vi "Write loopTimer.vi"(8 "error in (no error)":errorcluster, 10 "ILoopTimer.lvclass":refnum<class "ILoopTimer.lvclass">, 11 "WindowsTarget in":refnum<class "WindowsTarget.lvclass">) -> (0 "error out":errorcluster, 3 "WindowsTarget out":refnum<class "WindowsTarget.lvclass">)   [LabVIEW 2015, in "WindowsTarget.lvclass"]
uses:
  WindowsTarget.lvclass
  ComponentTemplateCore/ComponentModel/ComponentModelRT/LoopTimer/ILoopTimer/ILoopTimer.lvclass
  WindowsTarget.lvclass/WindowsTarget.ctl
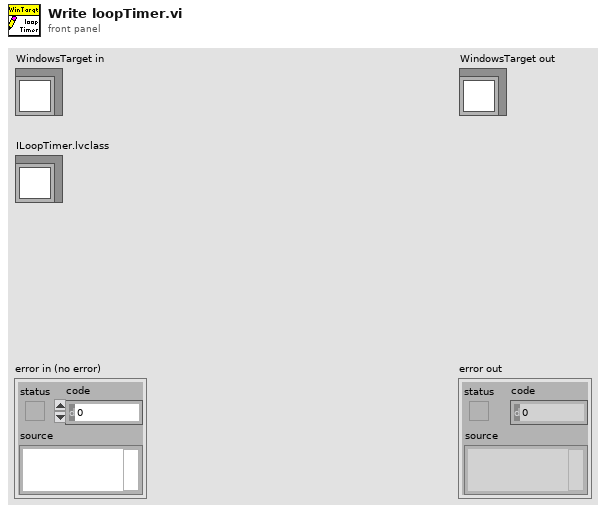
[diagram p1: front panel]
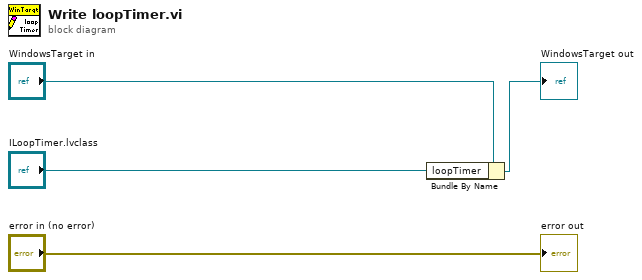
[diagram p0: block diagram]
diagram:
  n1 = Bundle By Name(cluster="WindowsTarget in", "loopTimer"="ILoopTimer.lvclass") -> (→"WindowsTarget out":refnum<class "WindowsTarget.lvclass">)
  "error out" <- "error in (no error)"
